vi "Populate Tree Item Children.vi"(11 "Type Tree In":T1[](array[typedef])) -> (3 "Type Tree":T1[](array[typedef]))   [LabVIEW 2018, in "LVClassByRef.lvlib"]
uses:
  <resource>/Framework/Providers/LVClassByRef/LVClassByRef.lvlib
  <resource>/Framework/Providers/LVClassByRef/Type Item.ctl
  <resource>/Framework/Providers/LVClassByRef/Tree Item.ctl
  <vilib>/Utility/Data Type/Type Definitions/Data Type.ctl
  <vilib>/Utility/Data Type/NI_Data Type.lvlib
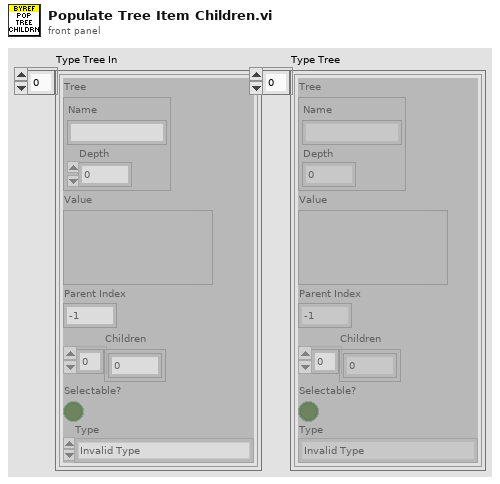
[diagram p1: front panel]
types:
  T1 = typedef "LVClassByRef.lvlib/Type Item.ctl" = cluster{"Tree":T2, "Value":variant, "Parent Index":i32, "Children":i32[], "Selectable?":bool, "Type":T3}
  T2 = typedef "LVClassByRef.lvlib/Tree Item.ctl" = cluster{"Name":string, "Depth":i32}
  T3 = typedef "NI_Data Type.lvlib/Data Type.ctl" = enum8{"Invalid Type", "Void", "I8", "I16", "I32", "I64", "U8", "U16", "U32", "U64", "Single Float", "Double Float", "Extended Float", "Single Complex", "Double Complex", "Extended Complex", "Enum U8", "Enum U16", "Enum U32", "Enum U64", "Single Float With Unit", "Double Float With Unit", "Extended Float With Unit", "Single Complex with Unit", "Double Complex with Unit", "Extended Complex with Unit", "Boolean", "String", "Path", "Picture", "Tag", "Array", "Cluster", "Variant", "LV Variant", "Waveform", "Timestamp", "Digital Waveform", "Digital Data", "ExpressData", "Refnum", "External Data", "VI", "Poly VI", "LabVIEW Class Instance", "Fixed Point"}
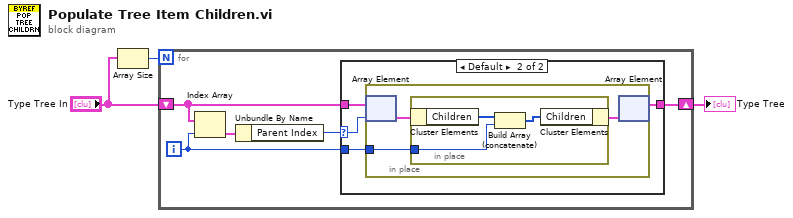
[diagram p0: block diagram]
diagram:
  n1 = Array Size(array="Type Tree In") -> (size(s)=w3:i32)
  n2 = for {
    N: w3 -> [_]
    shift-right: [w4] -> w1
    shift-left: "Type Tree In" -> [w7]
    i -> [w5]
    n3 = Index Array(array=w7, index=w5) -> (element=w8:T1)
    n4 = Unbundle By Name(w8) -> ("Parent Index"=w6:i32)
    n5 = case shown="Default" w6 {
      selector: w6 -> [_ w12]
      tunnel: w7 -> [w9 w13]
      tunnel: w5 -> [_ w11]
      tunnel: [w9 w10] -> w4
      frame -1 {
      }
      frame Default {
        n6 = in-place {
          in-place-border: w11 -> [w15]
          n7 = in-place-array #1(w13, w12) -> (w16:T1)
          n8 = in-place {
            in-place-border: w15 -> [w18]
            n9 = in-place-cluster #2(w16) -> ("Children"=w19:i32[])
            n10 = Build Array (concatenate)(w19, w18) -> (w17:i32[])
            n11 = in-place-cluster #2("Children"=w17) -> (w14:T1)
          }
          n12 = in-place-array #1(w14) -> (w10:T1[])  [unwired: 1 out]
        }
      }
    }
  }
  "Type Tree" <- w1
